vi "CursorDraw.vi"(8 "error in (no error)":errorcluster, 9 "Coords":T1, 11 "Gviewer in":refnum<class "Gviewer.lvclass">) -> (0 "error out":errorcluster, 3 "Gviewer out":refnum<class "Gviewer.lvclass">)   [LabVIEW 2020, in "Sgraph_lib_V1.lvlib" / "Gviewer.lvclass"]
doc: "Draw info at cursor point"
uses:
  Gviewer.lvclass
  <vilib>/Utility/miscctls.llb/LVPoint32TypeDef.ctl
  Gviewer.lvclass/Gviewer.ctl
  GV-ConvRangeGraph.vi
  GV-Layer-GT-zero.vi
  GV_CursorView.vi
  GV-LightenLineColor.vi
  GV-DrawYaxis.vi
  Common/controls/ToolTypeEnum.ctl
  Builds/Sgraph_lib_V1.lvlib
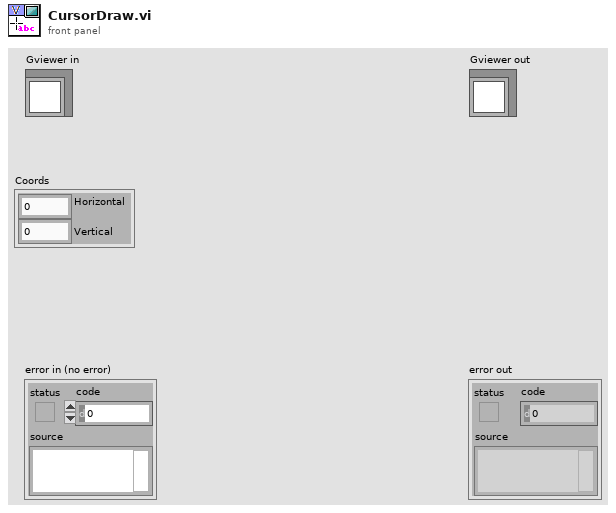
[diagram p1: front panel]
types:
  T1 = typedef "LVPoint32TypeDef.ctl" = cluster{"Horizontal":i32, "Vertical":i32}
  T2 = cluster{"horizontal":enum16{"left", "center", "right"}, "vertical":enum16{"top", "center", "bottom"}}
  T3 = typedef "LVRectTypeDef.ctl" = cluster{"Left":i16, "Top":i16, "Right":i16, "Bottom":i16}
  T4 = typedef "Sgraph_lib_V1.lvlib/Gviewer.lvclass/Typedef_SelProperties.ctl" = cluster{"Color":u32, "LineType":T5, "max":dbl, "min":dbl}
  T5 = typedef "Sgraph_lib_V1.lvlib/Gviewer.lvclass/Typedef_LineType.ctl" = enum16{"num_bare", "num_MinMax_Area", "num_MinMax_Lines", "num_MinMax_Forfor", "num_Max_Area", "num_Max_Line", "num_Max_Forfor", "num_Min_Area", "num_Min_Line", "num_Min_Fosfor", "Boolean_Line_01", "Boolean_Area_01", "Boolean_Fosfor_01", "Boolean_Line_TF", "Boolean_Area_TF", "Boolean_Fosfor_TF", "Boolean_OnOff_Line", "Boolean_OnOff_Area", "Boolean_OnOff_Fosfor", "Boolean_spare", "StringEvent_Line", "StringEvent_TimeLine"}
  T6 = typedef "Sgraph_lib_V1.lvlib/DBAL.lvclass/DBAL_TAGprops.ctl" = T7[]
  T7 = typedef "Sgraph_lib_V1.lvlib/DBAL.lvclass/DBAL_TAGpropEdit.ctl" = cluster{"TAG":string, "Qtype":string, "TAGprop":T8}
  T8 = typedef "Sgraph_lib_V1.lvlib/typedef_com_TagProp.ctl" = cluster{"Description":string, "EngUnits":string, "RangeH":dbl, "RangeL":dbl, "Resolution":i32, "Obsolete":bool, "ChangeDate":timestamp, "ChangeSource":string, "ChangeReason":string, "TagFunc":u32}
  T9 = typedef "Sgraph_lib_V1.lvlib/Gviewer.lvclass/Typedef_Live.ctl" = enum16{"Live View", "Freeze"}
  T10 = typedef "Sgraph_lib_V1.lvlib/FAMM.lvclass/FAMM_reply_datagram.ctl" = cluster{"GraphName":string, "Time-Start":timestamp, "Time-End":timestamp, "TimeSpan":dbl, "Live":T9, "WAQ_section":T11, "EAQ_section":T12, "PAQ_section":T13, "Layer":i32}
  T11 = typedef "Sgraph_lib_V1.lvlib/FAMM.lvclass/FAMM_reply_WAQdata.ctl" = cluster{"Boolean":bool}
  T12 = typedef "Sgraph_lib_V1.lvlib/FAMM.lvclass/FAMM_reply_EAQdata.ctl" = cluster{"Boolean":bool}
  T13 = typedef "Sgraph_lib_V1.lvlib/FAMM.lvclass/FAMM_reply_PAQdata.ctl" = cluster{"Tags":string[], "time stamp":timestamp[], "DataSection":cluster{"data":dbl[], "max":dbl[], "min":dbl[], "Status":u32[]}[]}
  T14 = typedef "Sgraph_lib_V1.lvlib/Gviewer.lvclass/LegendSet.ctl" = cluster{"Position":T15, "Size":T16, "Rows":u32, "Select":i32, "Visible":bool}
  T15 = typedef "LVPositionTypeDef.ctl" = cluster{"Left":i32, "Top":i32}
  T16 = typedef "LVBoundsTypeDef.ctl" = cluster{"Width":u32, "Height":u32}
  T17 = typedef "Sgraph_lib_V1.lvlib/ToolTypeEnum.ctl" = enum16{"00_Esc button", "01_Undo", "02_HelpButton", "03_CursorViewButton", "04_AutoScale_Fit", "05_AutoScale_Stacked", "06_ZoomWindowStart", "07_ZoomTimeStart", "08_ZoomAmplitudeStart", "09", "10", "11", "12", "13", "14", "15", "16", "17", "18", "19", "20_VerticalScroll", "21_VerticalMove", "22_TimeScroll", "23_TimeMove", "24", "25", "26_ZoomWindowSize", "27_ZoomTimeWindowSize", "28_ZoomAmplitudeWindowSize", "29", "30_LegendMovePoint", "31_LegendMoveDrag", "32", "33", "34", "35", "36", "37", "38", "39", "40_AddYscalePoint", "41_AddYscalePlace", "42_AddYscaleMovePoint", "43_AddYscaleMoveDrag", "44_AddYscaleDeletePoint"}
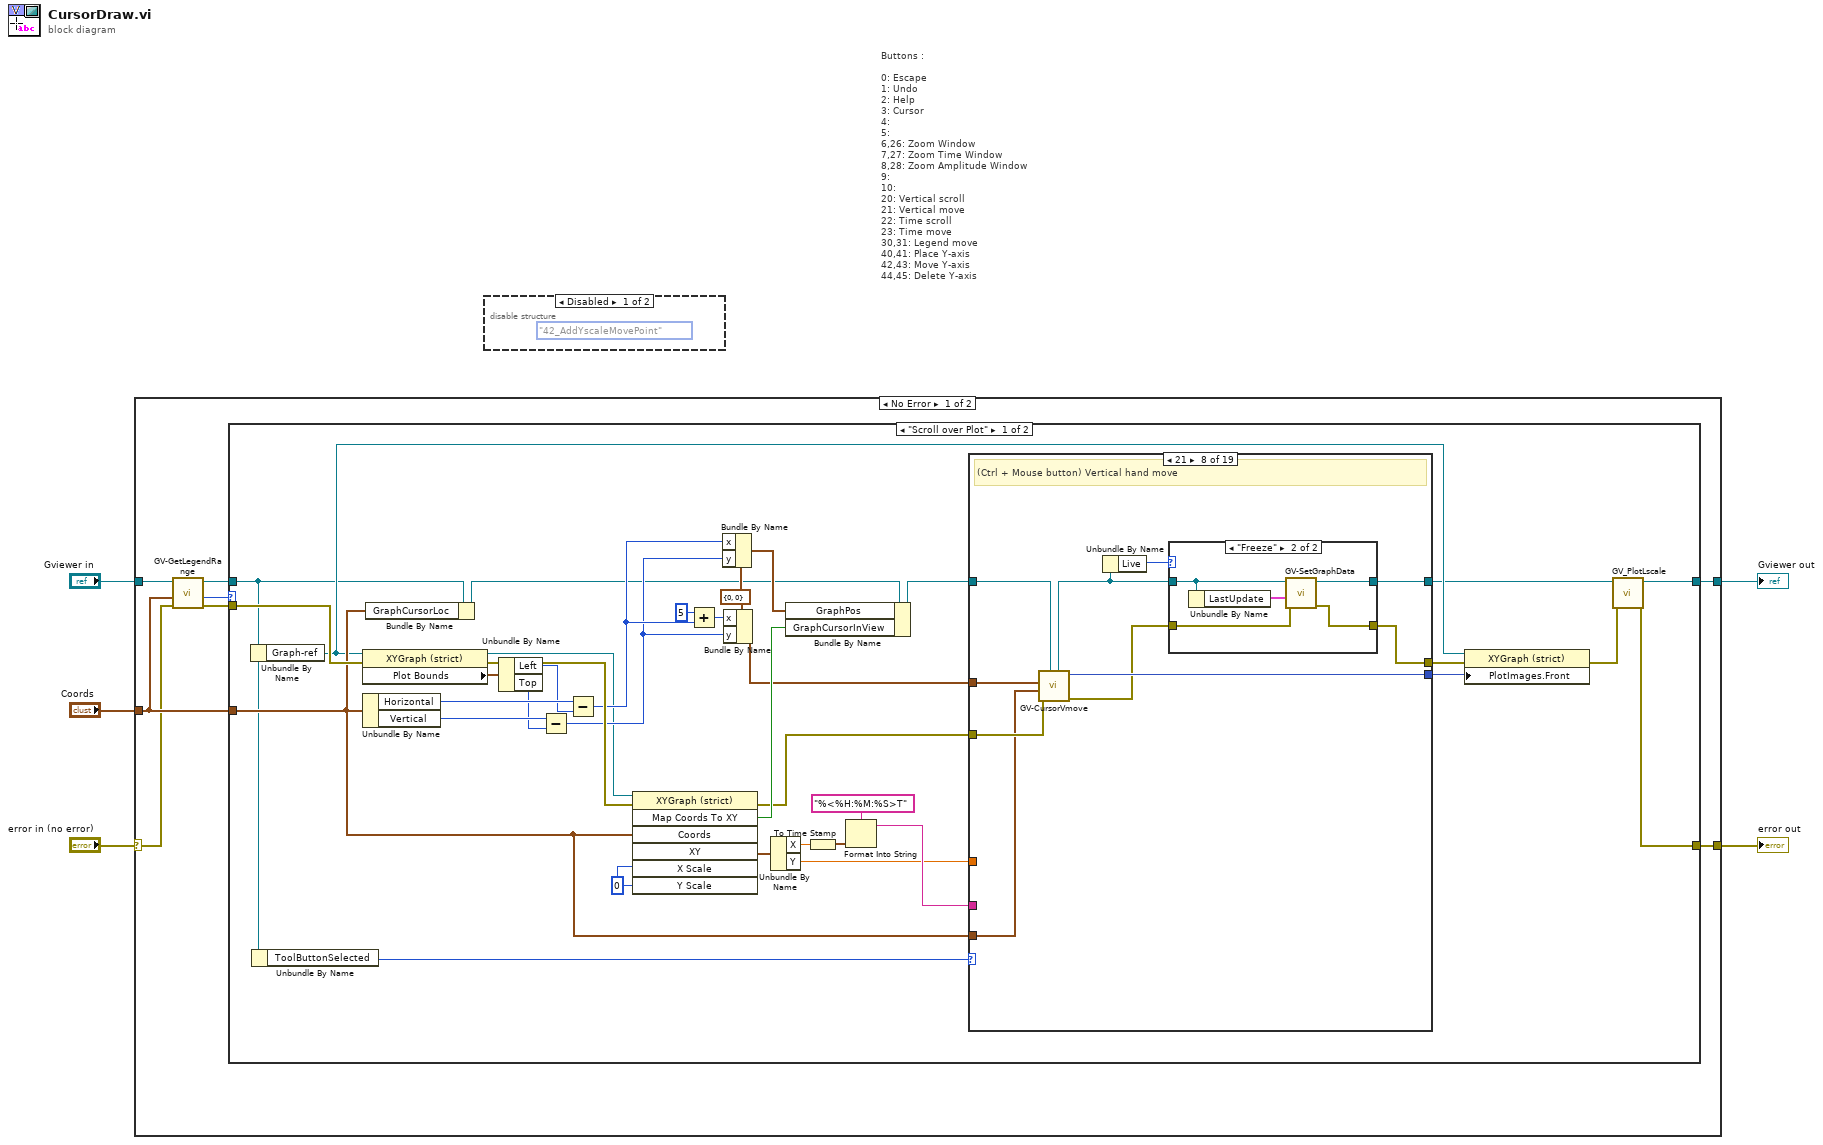
[diagram p0: block diagram]
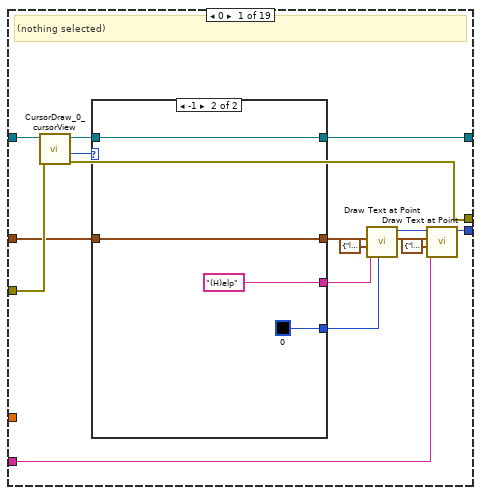
[diagram p3: hidden frame]
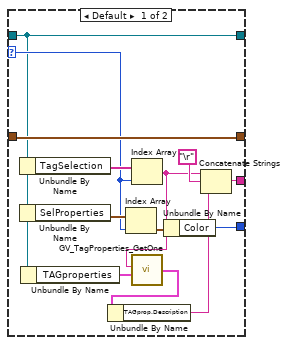
[diagram p4: hidden frame]
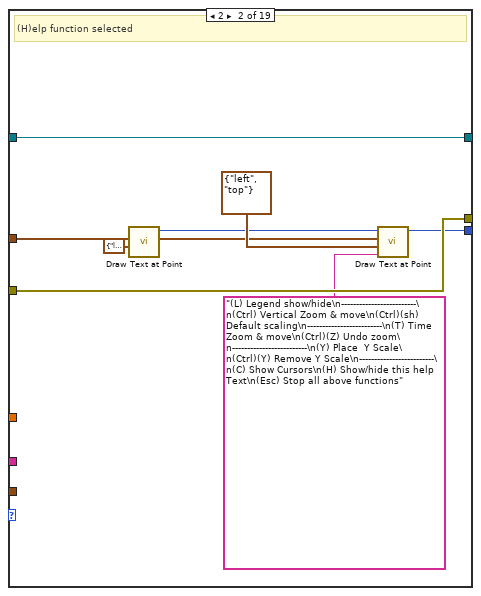
[diagram p5: hidden frame]
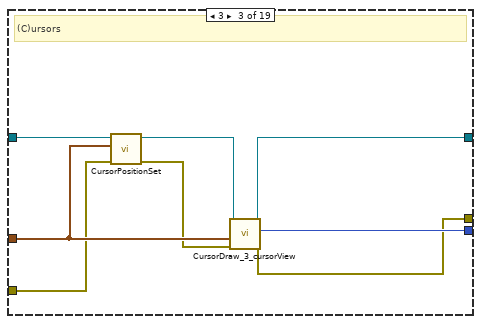
[diagram p6: hidden frame]
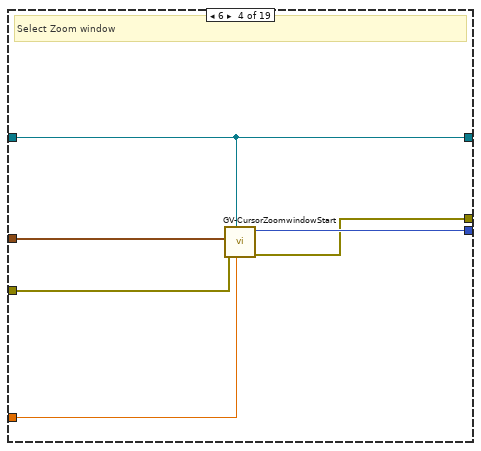
[diagram p7: hidden frame]
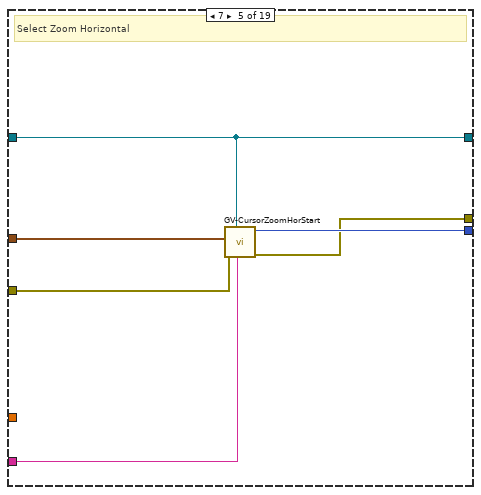
[diagram p8: hidden frame]
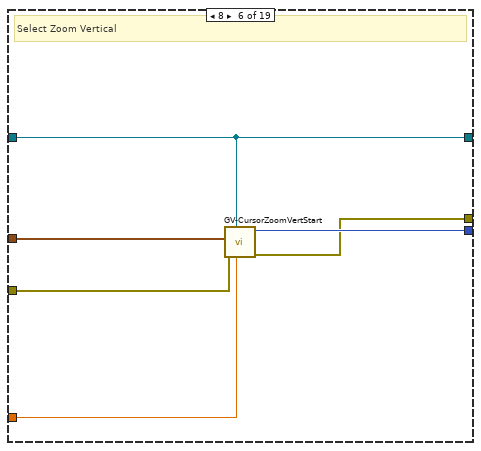
[diagram p9: hidden frame]
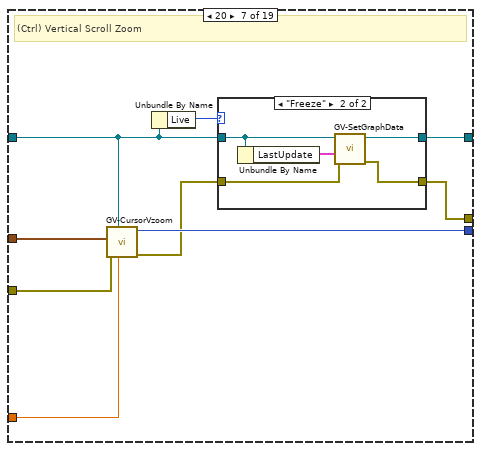
[diagram p10: hidden frame]
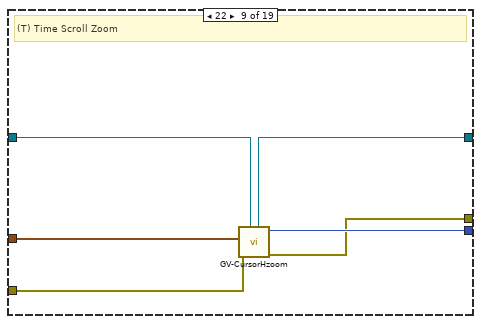
[diagram p13: hidden frame]
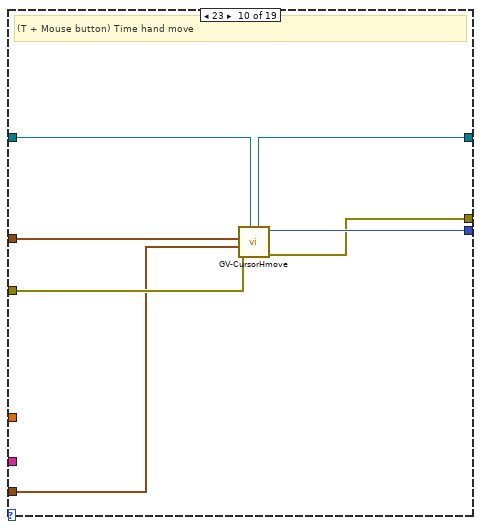
[diagram p14: hidden frame]
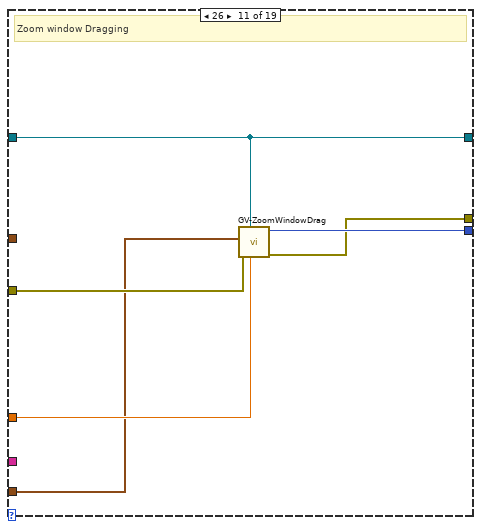
[diagram p15: hidden frame]
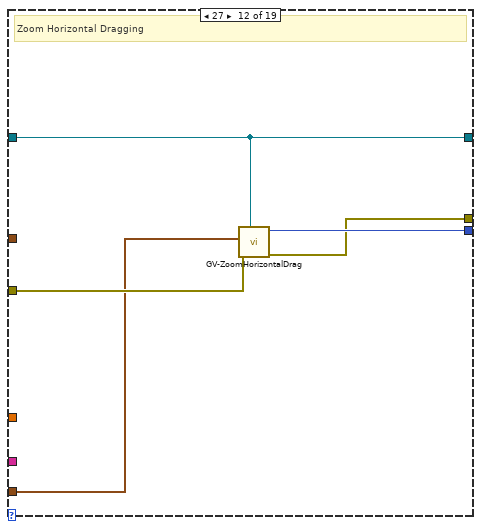
[diagram p16: hidden frame]
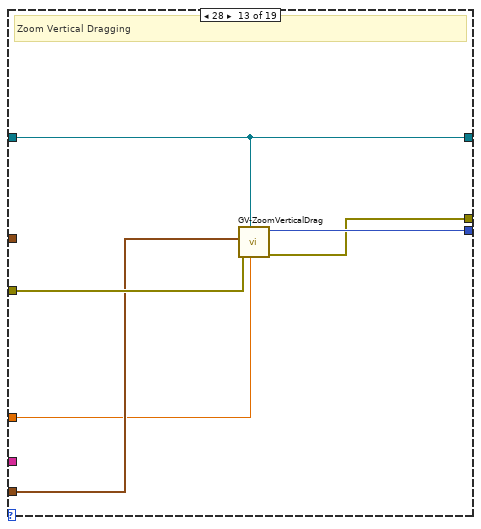
[diagram p17: hidden frame]
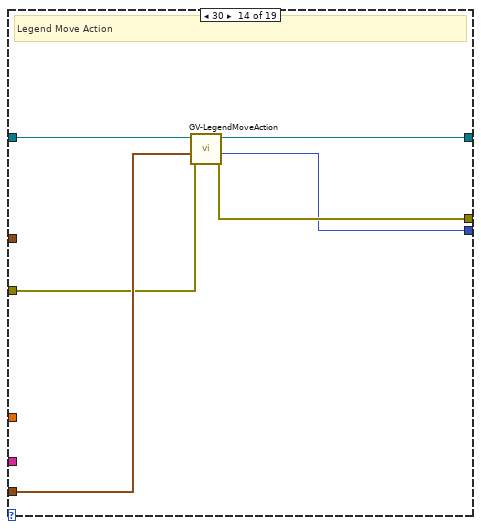
[diagram p18: hidden frame]
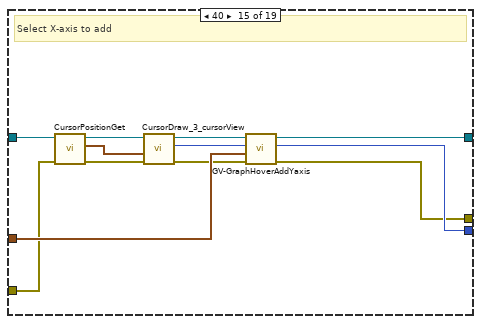
[diagram p19: hidden frame]
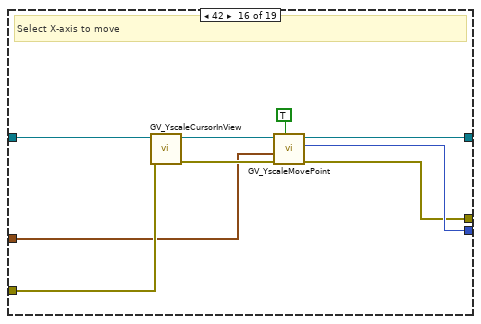
[diagram p20: hidden frame]
diagram:
  # "Buttons :\n\n0: Escape\n1: Undo\n2: Help\n3: Cursor\n4: \n5:\n6,26: Zoom Window\n7,27: Zoom Time Window\n8,28: Zoom Amplitude Window\n9:\n10:\n20: Vertical scroll\n21: Vertical move\n22: Time scroll\n23: Time move\n30,31: Legend move\n40,41: Place Y-axis\n42,43: Move Y-axis\n44,45: Delete Y-axis"
  n1 = case shown="No Error" "error in (no error)" {
    selector: "error in (no error)" -> [w6 w278]
    tunnel: [w12 w278] -> w4
    tunnel: [w13 w277] -> w2
    tunnel: "Gviewer in" -> [w10 w277]
    tunnel: "Coords" -> [w8 _]
    frame No Error {
      n2 = call "GV-GetLegendRange.vi"("error in (no error)"=w6, "Coords"=w8, "Gviewer in"=w10) -> ("error out"=w9:errorcluster, "Where?"=w7:enum16{"Scroll over Plot", "Scroll over Legend"}, "Gviewer out"=w11:refnum<class "Gviewer.lvclass">)  [unwired: 6 in]
      n3 = case shown="\"Scroll over Plot\"" w7 {
        tunnel: [w16 w227] -> w13
        tunnel: [w14 w228] -> w12
        tunnel: w11 -> [w18 w245]
        tunnel: w9 -> [w22 w230]
        tunnel: w8 -> [w21 w229]
        frame "Scroll over Plot" {
          w43 = 0 ("Y Scale")
          w31 = cluster{"x":i16, "y":i16} {"x"=0, "y"=0} ("origin")
          n4 = Unbundle By Name(w18) -> ("Graph-ref"=w19:refnum<vi>)
          n5 = Unbundle By Name(w18) -> ("ToolButtonSelected"=w26:i32)
          n6 = property class="XYGraph (strict)"(reference=w19, error in=w22) -> (reference out=w20:refnum<vi>, error out=w44:errorcluster, "Plot Bounds"=w49:T3)
          n7 = Unbundle By Name(w21) -> ("Horizontal"=w48:i32, "Vertical"=w47:i32)
          n8 = Bundle By Name(cluster=w18, "GraphCursorLoc"=w21) -> (w27:refnum<class "Gviewer.lvclass">)
          n9 = Unbundle By Name(w49) -> ("Left"=w46:i16, "Top"=w45:i16)
          n10 = Subtract(x=w47, y=w45) -> (x-y=w29:i32)
          n11 = Subtract(x=w48, y=w46) -> (x-y=w30:i32)
          n12 = invoke class="XYGraph (strict)" method="Map Coords To XY"(reference=w20, error in=w44, "Coords"=w21, "X Scale"=w43, "Y Scale"=w43) -> (error out=w33:errorcluster, "Map Coords To XY"=w41:bool, "XY"=w42:cluster{"X":dbl, "Y":dbl})  [unwired: 2 in, 4 out]
          n13 = Add(x=5, y=w30) -> (x+y=w36:i32)
          n14 = Bundle By Name(cluster=w31, "x"=w30, "y"=w29) -> (w28:cluster{"x":i16, "y":i16})
          n15 = Bundle By Name(cluster=w31, "x"=w36, "y"=w29) -> (w24:cluster{"x":i16, "y":i16})
          n16 = Unbundle By Name(w42) -> ("X"=w40:dbl, "Y"=w23:dbl)
          n17 = Bundle By Name(cluster=w27, "GraphPos"=w28, "GraphCursorInView"=w41) -> (w35:refnum<class "Gviewer.lvclass">)
          n18 = To Time Stamp(1:w40) -> (0:w39:timestamp)
          n19 = Format Into String(format string="%<%H:%M:%S>T", w39) -> (resulting string=w25:string)  [unwired: 2 in, 1 out]
          n20 = case shown="21" w26 {
            tunnel: w35 -> [w62 w89 w93 w99 w105 w111 w117 w139 w149 w155 w164 w169 w175 w184 w188 w205 w214 w220 w226]
            tunnel: [w59 w87 w97 w103 w109 w115 w124 w137 w154 w161 w167 w172 w178 w179 w193 w203 w212 w216 w223] -> w34
            tunnel: [w53 w89 w95 w99 w105 w111 w120 w134 w150 w156 w164 w169 w175 w182 w190 w202 w211 w217 w226] -> w17
            tunnel: w33 -> [w61 w88 w90 w102 w108 w114 w123 w141 w152 w159 w165 w170 w176 w181 w185 w200 w209 w219 w225]
            tunnel: [w60 w88 w96 w101 w107 w113 w118 w132 w153 w160 w166 w171 w177 w180 w191 w199 w208 w218 w225] -> w32
            tunnel: w25 -> [w63 _ _ _ w104 _ _ _ _ _ _ _ _ _ _ _ _ _ w222]
            tunnel: w24 -> [w52 w82 w92 w100 w106 w112 w122 w138 w151 w158 _ _ _ _ w196 w198 w207 w215 w221]
            tunnel: w23 -> [_ _ _ w98 _ w110 w121 _ _ _ w163 _ w173 _ _ _ _ _ _]
            tunnel: w21 -> [_ _ _ _ _ _ _ w140 _ w157 w162 w168 w174 w183 _ _ _ _ _]
            frame 0 {
              # "(nothing selected)"
              n21 = call "CursorDraw_0_cursorView.vi"("error in (no error)"=w61, "Gviewer in"=w62) -> ("error out"=w60:errorcluster, "Focus"=w57:i32, "Gviewer out"=w54:refnum<class "Gviewer.lvclass">)  [unwired: 7 in]
              n22 = case shown="-1" w57 {
                selector: w57 -> [w72 _]
                tunnel: [w68 "(H)elp"] -> w55
                tunnel: w54 -> [w71 w79]
                tunnel: [w71 w79] -> w53
                tunnel: w52 -> [w77 w80]
                tunnel: [w77 w80] -> w51
                tunnel: [w73 u32 0] -> w50
                frame Default {
                  n23 = Unbundle By Name(w71) -> ("TagSelection"=w76:string[])
                  n24 = Unbundle By Name(w71) -> ("SelProperties"=w75:T4[])
                  n25 = Unbundle By Name(w71) -> ("TAGproperties"=w67:T6)
                  n26 = Index Array(array=w75, index=w72) -> (element=w74:T4)
                  n27 = Index Array(array=w76, index=w72) -> (element=w66:string)
                  n28 = call "GV_TagProperties_GetOne.vi"("TAG"=w66, "TAGproperties"=w67) -> ("TAGproperty"=w65:T7)  [unwired: 5 in]
                  n29 = Unbundle By Name(w65) -> ("TAGprop.Description"=w70:string)
                  n30 = Unbundle By Name(w74) -> ("Color"=w73:u32)
                  n31 = Concatenate Strings(w66, "\r", w70) -> (w68:string)
                }
                frame -1 {
                }
              }
              n32 = call <vilib>:"Draw Text at Point.vi"("text color(black)"=w50, "text"=w55, "alignment(left, top)"=T2 {"horizontal"=enum."left", "vertical"=enum."top"}, "origin"=w51) -> ("new picture"=w58:picture)  [unwired: 6 in, 1 out]
              n33 = call <vilib>:"Draw Text at Point.vi"("text"=w63, "alignment(left, top)"=T2 {"horizontal"=enum."left", "vertical"=enum."bottom"}, "origin"=w51, "picture"=w58) -> ("new picture"=w59:picture)  [unwired: 6 in, 1 out]
            }
            frame 2 {
              # "(H)elp function selected"
              n34 = call <vilib>:"Draw Text at Point.vi"("alignment(left, top)"=T2 {"horizontal"=enum."left", "vertical"=enum."bottom"}, "origin"=w82) -> ("new picture"=w83:picture)  [unwired: 8 in, 1 out]
              n35 = call <vilib>:"Draw Text at Point.vi"("text"="(L) Legend show/hide\n-------------------------\n(Ctrl) Vertical Zoom & move\n(Ctrl)(sh) Default scaling\n-------------------------\n(T) Time Zoom & move\n(Ctrl)(Z) Undo zoom\n-------------------------\n(Y) Place  Y Scale\n(Ctrl)(Y) Remove Y Scale\n-------------------------\n(C) Show Cursors\n(H) Show/hide this help Text\n(Esc) Stop all above functions", "alignment(left, top)"=T2 {"horizontal"=enum."left", "vertical"=enum."top"}, "origin"=w82, "picture"=w83) -> ("new picture"=w87:picture)  [unwired: 6 in, 1 out]
            }
            frame 3 {
              # "(C)ursors"
              n36 = call "CursorPositionSet.vi"("error in (no error)"=w90, "CursorPosition"=w92, "Gviewer in"=w93) -> ("error out"=w91:errorcluster, "Gviewer out"=w94:refnum<class "Gviewer.lvclass">)  [unwired: 7 in]
              n37 = call "CursorDraw_3_cursorView.vi"("error in (no error)"=w91, "Pos"=w92, "Gviewer in"=w94) -> ("error out"=w96:errorcluster, "pict out"=w97:picture, "Gviewer out"=w95:refnum<class "Gviewer.lvclass">)  [unwired: 6 in]
            }
            frame 6 {
              # "Select Zoom window"
              n38 = call "GV-CursorZoomwindowStart.vi"("Y"=w98, "Gviewer in"=w99, "error in (no error)"=w102, "Pos"=w100) -> ("error out"=w101:errorcluster, "pict out"=w103:picture)  [unwired: 6 in]
            }
            frame 7 {
              # "Select Zoom Horizontal"
              n39 = call "GV-CursorZoomHorStart.vi"("time"=w104, "Gviewer in"=w105, "error in (no error)"=w108, "Pos"=w106) -> ("error out"=w107:errorcluster, "pict out"=w109:picture)  [unwired: 6 in]
            }
            frame 8 {
              # "Select Zoom Vertical"
              n40 = call "GV-CursorZoomVertStart.vi"("Y"=w110, "Gviewer in"=w111, "error in (no error)"=w114, "Pos"=w112) -> ("error out"=w113:errorcluster, "pict out"=w115:picture)  [unwired: 6 in]
            }
            frame 20 {
              # "(Ctrl) Vertical Scroll Zoom"
              n41 = call "GV-CursorVzoom.vi"("Y"=w121, "Gviewer in"=w117, "error in (no error)"=w123, "Pos"=w122) -> ("error out"=w119:errorcluster, "pict out"=w124:picture)  [unwired: 6 in]
              n42 = Unbundle By Name(w117) -> ("Live"=w116:T9)
              n43 = case shown="\"Freeze\"" w116 {
                tunnel: [w126 w130] -> w120
                tunnel: w117 -> [w126 w129]
                tunnel: w119 -> [w125 w128]
                tunnel: [w125 w127] -> w118
                frame "Live View", Default {
                }
                frame "Freeze" {
                  n44 = Unbundle By Name(w129) -> ("LastUpdate"=w131:T10)
                  n45 = call "GV-SetGraphData.vi"("error in (no error)"=w128, "GviewerUpdate"=w131, "Gviewer in"=w129) -> ("error out"=w127:errorcluster, "Gviewer out"=w130:refnum<class "Gviewer.lvclass">)  [unwired: 7 in]
                }
              }
            }
            frame 21 {
              # "(Ctrl + Mouse button) Vertical hand move"
              n46 = call "GV-CursorVmove.vi"("Gviewer in"=w139, "error in (no error)"=w141, "New coordinate"=w140, "Pos"=w138) -> ("error out"=w133:errorcluster, "pict out"=w137:picture, "Gviewer out"=w135:refnum<class "Gviewer.lvclass">)  [unwired: 5 in]
              n47 = Unbundle By Name(w135) -> ("Live"=w136:T9)
              n48 = case shown="\"Freeze\"" w136 {
                tunnel: [w143 w147] -> w134
                tunnel: w135 -> [w143 w146]
                tunnel: w133 -> [w142 w145]
                tunnel: [w142 w144] -> w132
                frame "Live View", Default {
                }
                frame "Freeze" {
                  n49 = Unbundle By Name(w146) -> ("LastUpdate"=w148:T10)
                  n50 = call "GV-SetGraphData.vi"("error in (no error)"=w145, "GviewerUpdate"=w148, "Gviewer in"=w146) -> ("error out"=w144:errorcluster, "Gviewer out"=w147:refnum<class "Gviewer.lvclass">)  [unwired: 7 in]
                }
              }
            }
            frame 22 {
              # "(T) Time Scroll Zoom"
              n51 = call "GV-CursorHzoom.vi"("Gviewer in"=w149, "error in (no error)"=w152, "Pos"=w151) -> ("error out"=w153:errorcluster, "pict out"=w154:picture, "Gviewer out"=w150:refnum<class "Gviewer.lvclass">)  [unwired: 6 in]
            }
            frame 23 {
              # "(T + Mouse button) Time hand move"
              n52 = call "GV-CursorHmove.vi"("Gviewer in"=w155, "error in (no error)"=w159, "New coordinate"=w157, "Pos"=w158) -> ("error out"=w160:errorcluster, "pict out"=w161:picture, "Gviewer out"=w156:refnum<class "Gviewer.lvclass">)  [unwired: 5 in]
            }
            frame 26 {
              # "Zoom window Dragging"
              n53 = call "GV-ZoomWindowDrag.vi"("Y"=w163, "Gviewer in"=w164, "error in (no error)"=w165, "Coords"=w162) -> ("error out"=w166:errorcluster, "pict out"=w167:picture)  [unwired: 6 in]
            }
            frame 27 {
              # "Zoom Horizontal Dragging"
              n54 = call "GV-ZoomHorizontalDrag.vi"("Gviewer in"=w169, "error in (no error)"=w170, "Coords"=w168) -> ("error out"=w171:errorcluster, "pict out"=w172:picture)  [unwired: 7 in]
            }
            frame 28 {
              # "Zoom Vertical Dragging"
              n55 = call "GV-ZoomVerticalDrag.vi"("Y"=w173, "Gviewer in"=w175, "error in (no error)"=w176, "Coords"=w174) -> ("error out"=w177:errorcluster, "pict out"=w178:picture)  [unwired: 6 in]
            }
            frame 30 {
              # "Legend Move Action"
              n56 = call "GV-LegendMoveAction.vi"("error in (no error)"=w181, "Coords"=w183, "Gviewer in"=w184) -> ("error out"=w180:errorcluster, "Plot Images:Front"=w179:picture, "Gviewer out"=w182:refnum<class "Gviewer.lvclass">)  [unwired: 6 in]
            }
            frame 40 {
              # "Select X-axis to add"
              n57 = call "CursorPositionGet.vi"("error in (no error)"=w185, "Gviewer in"=w188) -> ("error out"=w186:errorcluster, "CursorPosition"=w187:cluster{"x":i16, "y":i16}, "Gviewer out"=w189:refnum<class "Gviewer.lvclass">)  [unwired: 7 in]
              n58 = call "CursorDraw_3_cursorView.vi"("error in (no error)"=w186, "Pos"=w187, "Gviewer in"=w189) -> ("error out"=w192:errorcluster, "pict out"=w194:picture, "Gviewer out"=w195:refnum<class "Gviewer.lvclass">)  [unwired: 6 in]
              n59 = call "GV-GraphHoverAddYaxis.vi"("error in (no error)"=w192, "Pos"=w196, "Plot in"=w194, "Gviewer in"=w195) -> ("error out"=w191:errorcluster, "Plot out"=w193:picture, "Gviewer out"=w190:refnum<class "Gviewer.lvclass">)  [unwired: 5 in]
            }
            frame 42 {
              # "Select X-axis to move"
              n60 = call "GV_YscaleCursorInView.vi"("error in (no error)"=w200, "Gviewer in"=w205) -> ("error out"=w201:errorcluster, "Gviewer out"=w204:refnum<class "Gviewer.lvclass">)  [unwired: 8 in]
              n61 = call "GV_YscaleMovePoint.vi"("Move?"=TRUE, "error in (no error)"=w201, "Pos"=w198, "Gviewer in"=w204) -> ("error out"=w199:errorcluster, "Plot out"=w203:picture, "Gviewer out"=w202:refnum<class "Gviewer.lvclass">)  [unwired: 5 in]
            }
            frame 44 {
              # "Select X-axis to delete"
              n62 = call "GV_YscaleCursorInView.vi"("error in (no error)"=w209, "Gviewer in"=w214) -> ("error out"=w210:errorcluster, "Gviewer out"=w213:refnum<class "Gviewer.lvclass">)  [unwired: 8 in]
              n63 = call "GV_YscaleDeletePoint.vi"("Move?"=TRUE, "error in (no error)"=w210, "Pos"=w207, "Gviewer in"=w213) -> ("error out"=w208:errorcluster, "Plot out"=w212:picture, "Gviewer out"=w211:refnum<class "Gviewer.lvclass">)  [unwired: 5 in]
            }
            frame 41, 43 {
              # "Set location of Yaxis to place"
              n64 = call "GV_YscaleLocatePlace.vi"("error in (no error)"=w219, "Pos"=w215, "Gviewer in"=w220) -> ("error out"=w218:errorcluster, "Plot Images:Front"=w216:picture, "Gviewer out"=w217:refnum<class "Gviewer.lvclass">)  [unwired: 6 in]
            }
            frame Default {
              # "Standard (ESC) time only"
              n65 = call <vilib>:"Draw Text at Point.vi"("text"=w222, "alignment(left, top)"=T2 {"horizontal"=enum."left", "vertical"=enum."bottom"}, "origin"=w221) -> ("new picture"=w223:picture)  [unwired: 7 in, 1 out]
            }
          }
          n66 = property class="XYGraph (strict)"(reference=w19, error in=w32, "PlotImages.Front"=w34) -> (error out=w15:errorcluster)  [unwired: 1 out]
          n67 = call "GV_PlotLscale.vi"("error in (no error)"=w15, "Gviewer in"=w17) -> ("error out"=w14:errorcluster, "Gviewer out"=w16:refnum<class "Gviewer.lvclass">)  [unwired: 8 in]
        }
        frame "Scroll over Legend" {
          w253 = 5  # Border width
          n68 = Unbundle By Name(w245) -> ("Graph-ref"=w242:refnum<vi>)
          n69 = Unbundle By Name(w229) -> ("Horizontal"=w240:i32, "Vertical"=w239:i32)
          n70 = Unbundle By Name(w245) -> ("Left"=w260:i32, "Top"=w252:i32, "Width"=w259:u32, "Height"=w256:u32)
          n71 = property class="XYGraph (strict)"(reference=w242, error in=w230) -> (reference out=w237:refnum<vi>, error out=w231:errorcluster, "Plot Bounds"=w241:T3)
          n72 = Add(x=w260, y=w259) -> (x+y=w258:u32)
          n73 = Add(x=w256, y=w252) -> (x+y=w255:u32)
          n74 = Unbundle By Name(w241) -> ("Left"=w235:i16, "Top"=w233:i16)
          n75 = Negate(x=w235) -> (-x=w234:i16)
          n76 = Negate(x=w233) -> (-x=w232:i16)
          n77 = Subtract(x=w255, y=w253) -> (x-y=w254:u32)
          n78 = Add(x=w253, y=w252) -> (x+y=w251:i32)
          n79 = Add(x=w253, y=w260) -> (x+y=w261:i32)
          n80 = Subtract(x=w258, y=w253) -> (x-y=w257:u32)
          n81 = Bundle By Name(cluster=cluster{"x":i16, "y":i16} {"x"=0, "y"=0}, "x"=w234, "y"=w232) -> (w236:cluster{"x":i16, "y":i16})
          n82 = In Range and Coerce(upper limit=w261, x=w240, lower limit=w260) -> (In Range?=w250:bool)  [unwired: 1 out]
          n83 = In Range and Coerce(upper limit=w258, x=w240, lower limit=w257) -> (In Range?=w247:bool)  [unwired: 1 out]
          n84 = In Range and Coerce(upper limit=w255, x=w239, lower limit=w254) -> (In Range?=w248:bool)  [unwired: 1 out]
          n85 = In Range and Coerce(upper limit=w251, x=w239, lower limit=w252) -> (In Range?=w249:bool)  [unwired: 1 out]
          n86 = Compound Arithmetic op=OR "or"(w250, w247, w248, w249) -> (w246:bool)
          n87 = case shown="True" w246 {
            tunnel: w245 -> [w268 w270]
            tunnel: w231 -> [w266 w276]
            tunnel: [w267 w271] -> w227
            tunnel: [w265 w276] -> w244
            tunnel: [w263 w274] -> w243
            tunnel: w236 -> [w262 w273]
            tunnel: w229 -> [w264 _]
            frame False {
              # "Mouse over TAG area"
              n88 = call "GV-LegendMouseOver.vi"("Origin"=w262, "error in (no error)"=w266, "Coords"=w264, "Gviewer in"=w268) -> ("error out"=w265:errorcluster, "image"=w263:picture, "Gviewer out"=w267:refnum<class "Gviewer.lvclass">)  [unwired: 5 in]
            }
            frame True {
              # "Mouse over move Area"
              n89 = Bundle By Name(cluster=w270, "Select"=-2 ("Legend.Select")) -> (w271:refnum<class "Gviewer.lvclass">)
              n90 = Unbundle By Name(w271) -> ("Legend"=w275:T14)
              n91 = call "GV_Legend_DrawMove.vi"("Legend"=w275, "Select"=FALSE, "Origin"=w273) -> ("Image"=w274:picture)  [unwired: 6 in]
            }
          }
          n92 = property class="XYGraph (strict)"(reference=w237, error in=w244, "PlotImages.Front"=w243) -> (error out=w228:errorcluster)  [unwired: 1 out]
        }
      }
    }
    frame Error {
    }
  }
  "error out" <- w4
  "Gviewer out" <- w2
  n93 = disable-structure shown="Disabled" {
    frame Disabled {
      (unwired) ToolTypeEnum."42_AddYscaleMovePoint" ("Enum")
    }
    frame Enabled {
    }
  }
